vi "Der_b.vi"(1 "dZ_l":T1, 2 "m":dbl) -> (0 "db_l":T1)   [LabVIEW 2016]
uses:
  <vilib>/Analysis/Matrix/Datatypes/RealMatrix.ctl
  <vilib>/Analysis/Matrix/Numeric/Conversions/Array To Matrix - RA2.vi
  <vilib>/Analysis/Matrix/NI_Matrix.lvlib
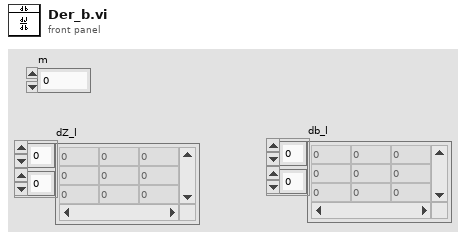
[diagram p1: front panel]
types:
  T1 = typedef "NI_Matrix.lvlib/RealMatrix.ctl" = dbl[][]
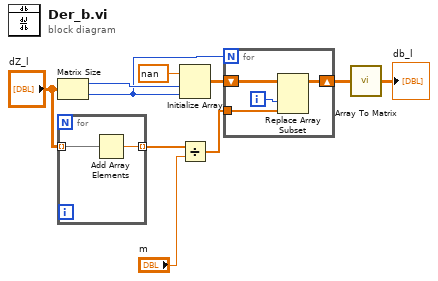
[diagram p0: block diagram]
diagram:
  n1 = Matrix Size(0:"dZ_l") -> (1:w6:i32, 2:w5:i32)
  n2 = for {
    tunnel: "dZ_l" -> [w12] mode=indexing
    tunnel: [w11] -> w9 mode=indexing
    n3 = Add Array Elements(numeric array=w12) -> (sum=w11:dbl)
  }
  n4 = Initialize Array(nan ("element"), w6, w5) -> (w4:dbl[][])
  n5 = Divide(x=w9, y="m") -> (x/y=w3:dbl[])
  n6 = for {
    N: w5 -> [_]
    shift-right: [w15] -> w2
    shift-left: w4 -> [w16]
    tunnel: w3 -> [w14]
    i -> [w13]
    n7 = Replace Array Subset(array=w16, new element=w14, index (col)=w13) -> (w15:dbl[][])  [unwired: 1 in]
  }
  n8 = call-poly <vilib>:"Array To Matrix.vi"("Real 2D Array"=w2) -> ("Real Matrix"=→"db_l":T1)
